vi "DIGitize.vi"(8 "Error":errorcluster caption="错误输入（无错误）", 10 "Channel":u32, 11 "VISA resource name":refnum<visa-resource-name>) -> (0 "Error out":errorcluster, 3 "VISA resource name out":refnum<visa-resource-name>)   [LabVIEW 2020]
doc: "采集完成后停止"
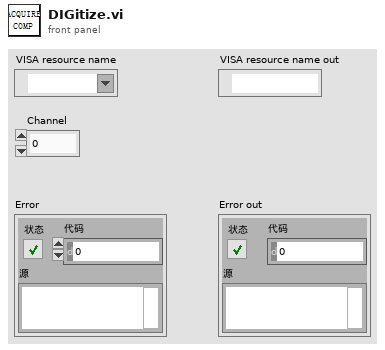
[diagram p1: front panel]
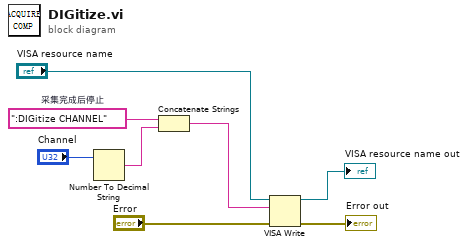
[diagram p0: block diagram]
diagram:
  w7 = ":DIGitize CHANNEL"  # 采集完成后停止
  n1 = Number To Decimal String(number="Channel") -> (decimal integer string=w5:string)  [unwired: 1 in]
  n2 = Concatenate Strings(w7, w5) -> (w1:string)
  n3 = VISA Write(VISA resource name="VISA resource name", write buffer=w1, error in (no error)="Error") -> (VISA resource name out=→"VISA resource name out":refnum<visa-resource-name>, error out=→"Error out":errorcluster)  [unwired: 1 out]
